vi "Milliseconds to Minutes Seconds.vi"(11 "milliseconds":u32) -> (3 "minutes:seconds":string)   [LabVIEW 2020, in "Template Tool.lvlib"]
uses:
  Template Tool.lvlib
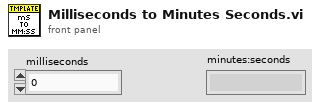
[diagram p1: front panel]
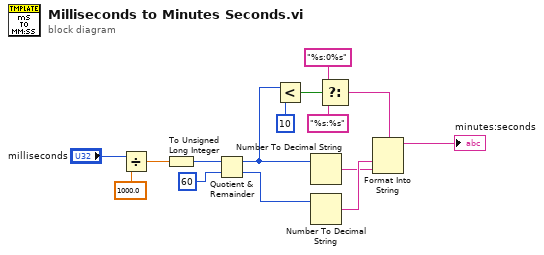
[diagram p0: block diagram]
diagram:
  n1 = Divide(x="milliseconds", y=1000.0) -> (x/y=w9:dbl)
  n2 = To Unsigned Long Integer(number=w9) -> (unsigned 32bit integer=w7:u32)
  n3 = Quotient & Remainder(x=w7, y=u32 60 ("milliseconds")) -> (x-y*floor(x/y)=w6:u32, floor(x/y)=w13:u32)
  n4 = Less?(x=w6, y=u32 10 ("milliseconds")) -> (x < y?=w4:bool)
  n5 = Number To Decimal String(number=w6) -> (decimal integer string=w10:string)  [unwired: 1 in]
  n6 = Number To Decimal String(number=w13) -> (decimal integer string=w12:string)  [unwired: 1 in]
  n7 = Select(t="%s:0%s" ("format string"), s=w4, f="%s:%s" ("format string")) -> (s? t:f=w3:string)
  n8 = Format Into String(format string=w3, w12, w10) -> (resulting string=→"minutes:seconds":string)  [unwired: 2 in, 1 out]
